vi "Select host address.vi"(0 "System number":i32=1 min=1 max=4 step=1, 1 "Port":i32=50000, 2 "Controller names":string[](array[string]), 3 "Mode":T1(ring), 4 "All?":bool, 5 "error in":errorcluster) -> (14 "Selected Host address/name":string="localhost", 15 "Port out":i32=50000, 19 "error out":errorcluster)   [LabVIEW 2026]
doc: "Performs an UDP broadcast, returns IP addresses and names of all controllers matching Controller name and lets the user select the appropriate controller from a ring control. VI will also stop if Cancel is TRUE.\n\nC-413: Controller names = C-413, Mode = Find XPort by UDP, Port = 30718\nC-413: Controller names = C-413, Mode = Find USR-K3 by UDP, Port = 1901\nC-702: Controller names = C-702, Mode = Find controller by UDP, Port = 50000 \nC-867: Controller names = C-867, Mode = Find controller by UDP, Port = 50000\nC-884: Controller names = C-884, Mode = Find controller by UDP, Port = 50000\nC-885: Controller names = C-885, Mode = Find controller by UDP, Port = 50000\nC-886: Controller names = C-886, Mode = Find controller by UDP, Port = 50000\nC-891: Controller names = C-891, Mode = Find XPort by UDP, Port = 30718\nE-135: Controller names = E-135, Mode = Find USR-K3 by UDP, Port = 1901\nE-517: Controller names = E-517, Mode = Find controller by UDP, Port = 50000\nE-518: Controller names = E-518, Mode = Find controller by UDP, Port = 50000\nE-712: Controller names = E-712, Mode = Find controller by UDP, Port = 50000\nE-725: Controller names = E-725, Mode = Find XPort by UDP, Port = 30718\nE-725: Controller names = E-725, Mode = Find controller by UDP, Port = 50000\nE-753: Controller names = E-753, Mode = Find controller by UDP, Port = 50000\nE-754: Controller names = E-754, Mode = Find controller by UDP, Port = 50000\nE-871: Controller names = E-871, Mode = Find XPort by UDP, Port = 30718\nE-872: Controller names = E-872, Mode = Find controller by UDP, Port = 50000\nE-873: Controller names = E-873, Mode = Find XPort by UDP, Port = 30718\nE-874: Controller names = E-874, Mode = Find USR-K3 by UDP, Port = 1901\nF-206: Controller names = F-206, F-HEX, Mode = Find XPort by UDP, Port = 30718\nC-887, M-8X0: Controller names = M-8X0, HEXAPOD, Mode = Find XPort by UDP, Port = 30718"
panel:
  in  "abort":bool
  in  "ok":bool
  in  "Please select controller":u16(ring) items=["(c)2013-2015 Physik Instrumente (PI) GmbH & Co. KG,C-413K006,0155500004,0.011 -- listening on port 2000 -- at address: 172.16.50.50"]
  out "Please wait":string="Broadcast is running, please wait..."
  # "Port to scan and controller name to search for:"
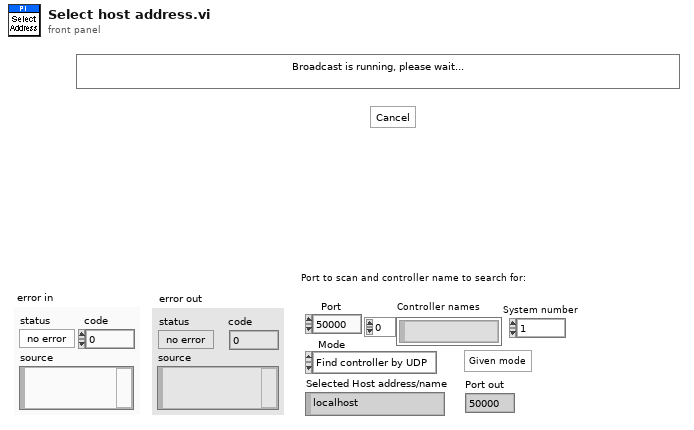
[diagram p1: front panel]
types:
  T1 = enum16{"Find controller by UDP", "Find XPort by UDP", "Find USR-K3 by UDP"}
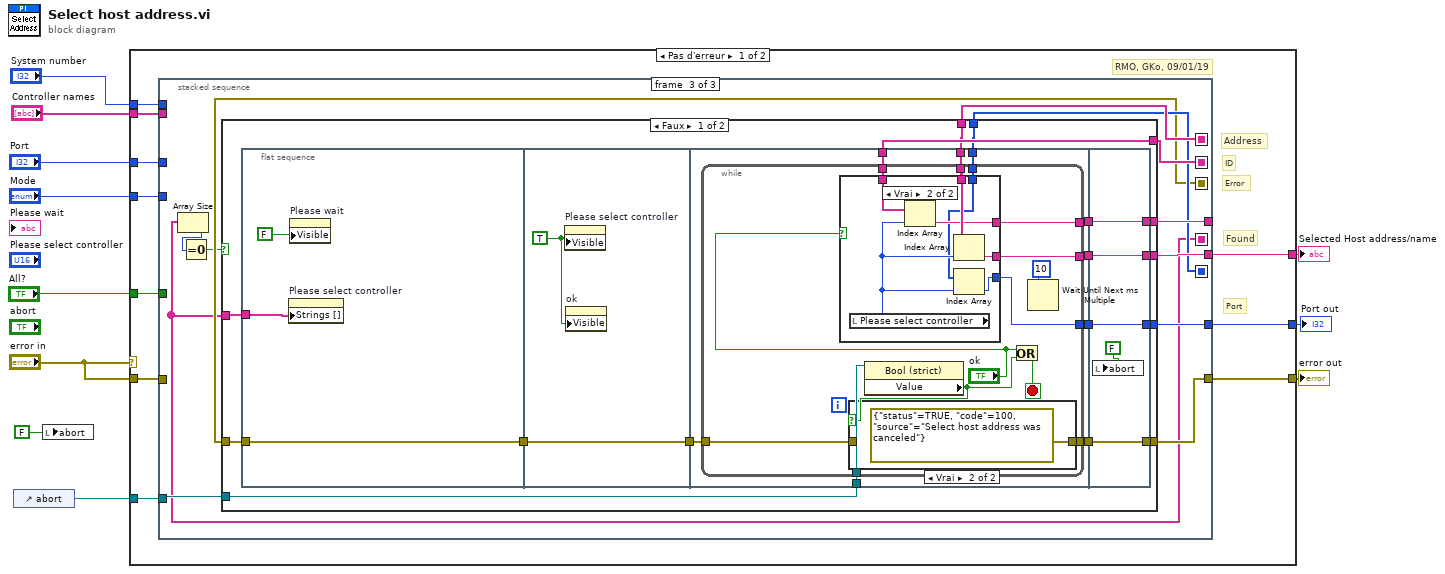
[diagram p0: block diagram]
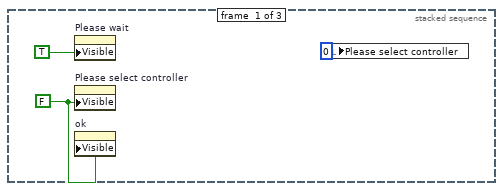
[diagram p2: hidden frame]
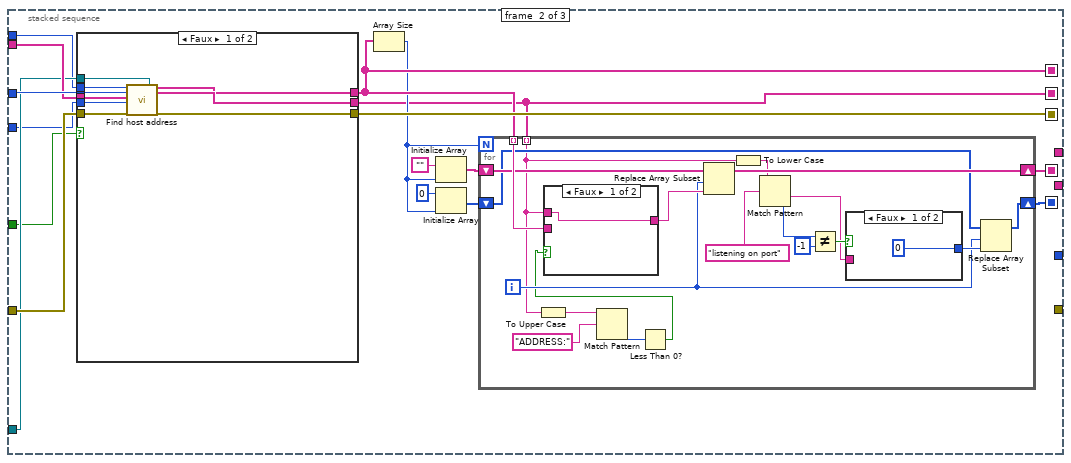
[diagram p3: hidden frame]
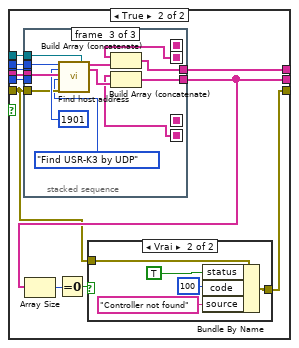
[diagram p4: hidden frame]
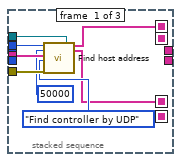
[diagram p6: hidden frame]
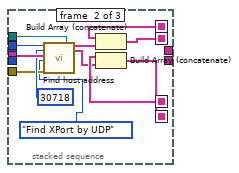
[diagram p7: hidden frame]
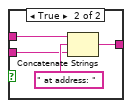
[diagram p8: hidden frame]
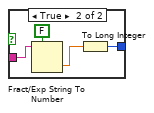
[diagram p9: hidden frame]
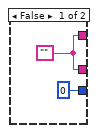
[diagram p11: hidden frame]
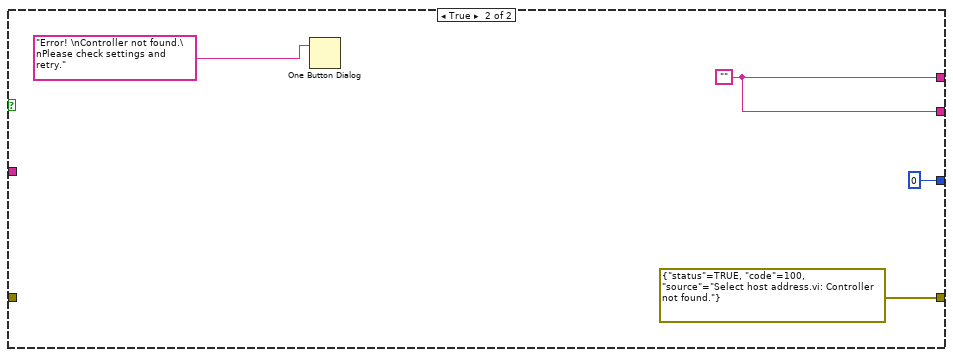
[diagram p12: hidden frame]
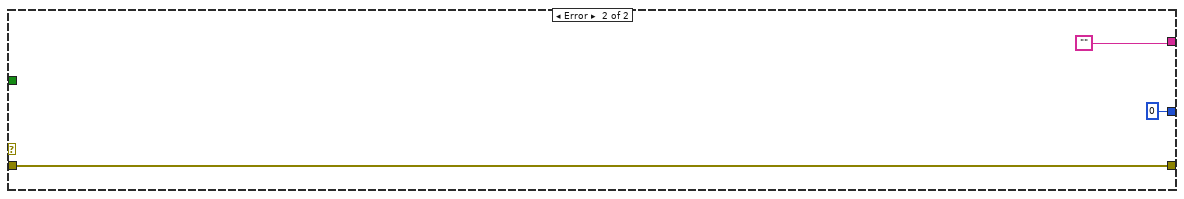
[diagram p13: hidden frame]
diagram:
  n1 = control-ref of="abort"() -> (w8:refnum<vi>)
  n2 = local write "abort"(FALSE ("abort")) -> ()
  n3 = case shown="Pas d'erreur" "error in" {
    tunnel: [w18 w206] -> w11
    tunnel: "error in" -> [w19 w206]
    tunnel: "Port" -> [w21 _]
    tunnel: "Controller names" -> [w20 _]
    tunnel: w8 -> [w17 _]
    tunnel: [w15 "" ("Host address/name")] -> w7
    tunnel: "Mode" -> [w16 _]
    tunnel: [w14 0] -> w5
    tunnel: "System number" -> [w13 _]
    tunnel: "All?" -> [w12 _]
    frame No Error {
      # "Port"
      # "Error"
      # "Found"
      # "Address"
      # "ID"
      # "RMO, GKo, 09/01/19"
      n4 = stacked-sequence {
        seq-local: [_ w36 _] -> [_ _ w133]
        seq-local: [_ w35 _] -> [_ _ w131]
        seq-local: [_ w34 _] -> [_ _ w139]
        seq-local: [_ w25 _] -> [_ _ w140]
        seq-local: [_ w28 _] -> [_ _ w135]
        tunnel: w21 -> [_ w41 _]
        tunnel: w20 -> [_ w40 _]
        tunnel: w19 -> [_ w39 _]
        tunnel: [_ _ w132] -> w18
        tunnel: [_ _ w138] -> _
        tunnel: [_ _ w137] -> w15
        tunnel: w17 -> [_ w33 w136]
        tunnel: w16 -> [_ w32 _]
        tunnel: [_ _ w134] -> w14
        tunnel: w13 -> [_ w27 _]
        tunnel: w12 -> [_ w26 _]
        frame #0 {
          w23 = FALSE ("Visible")
          n5 = property on="Please wait" class="Ch"("Visible"=TRUE) -> ()  [unwired: 2 in, 2 out]
          n6 = property on="Please select controller" class="MDér (strict)"("Visible"=w23) -> ()  [unwired: 2 in, 2 out]
          n7 = property on="ok" class="Bool"("Visible"=w23) -> ()  [unwired: 2 in, 2 out]
          n8 = local write "Please select controller"(0) -> ()
        }
        frame #1 {
          n9 = case shown="Faux" w26 {
            tunnel: w41 -> [w50 w61]
            tunnel: w40 -> [w49 w60]
            tunnel: w39 -> [w48 w51]
            tunnel: [w47 w53] -> w36
            tunnel: [w46 w52] -> w25
            tunnel: [w45 w59] -> w34
            tunnel: w33 -> [w44 w58]
            tunnel: w32 -> [w43 w57]
            tunnel: w27 -> [w42 w56]
            frame False {
              n10 = call "Find host address.vi"("System number"=w42, "Port"=w50, "Controller names"=w49, "Mode"=w43, "error in"=w48, "Stop refnum"=w44) -> ("Address"=w45:string[], "ID"=w46:string[], "error out"=w47:errorcluster)  [unwired: 11 out]
            }
            frame True {
              n11 = stacked-sequence {
                seq-local: [w69 _ _] -> [_ w83 _]
                seq-local: [w68 _ _] -> [_ w81 _]
                seq-local: [_ w79 _] -> [_ _ w92]
                seq-local: [_ w78 _] -> [_ _ w91]
                tunnel: w61 -> [_ _ _]
                tunnel: w60 -> [w75 w87 w99]
                tunnel: w51 -> [w74 w77 w89]
                tunnel: [_ _ w90] -> w52
                tunnel: [_ _ w94] -> w59
                tunnel: w58 -> [w73 w86 w98]
                tunnel: w57 -> [_ _ _]
                tunnel: w56 -> [w72 w85 w97]
                frame #0 {
                  n12 = call "Find host address.vi"("System number"=w72, "Port"=50000, "Controller names"=w75, "Mode"=T1."Find controller by UDP", "error in"=w74, "Stop refnum"=w73) -> ("Address"=w69:string[], "ID"=w68:string[])  [unwired: 12 out]
                }
                frame #1 {
                  n13 = call "Find host address.vi"("System number"=w85, "Port"=30718, "Controller names"=w87, "Mode"=T1."Find XPort by UDP", "error in"=w77, "Stop refnum"=w86) -> ("Address"=w82:string[], "ID"=w80:string[])  [unwired: 12 out]
                  n14 = Build Array (concatenate)(w83, w82) -> (w79:string[])
                  n15 = Build Array (concatenate)(w81, w80) -> (w78:string[])
                }
                frame #2 {
                  n16 = call "Find host address.vi"("System number"=w97, "Port"=1901, "Controller names"=w99, "Mode"=T1."Find USR-K3 by UDP", "error in"=w89, "Stop refnum"=w98) -> ("Address"=w95:string[], "ID"=w93:string[])  [unwired: 12 out]
                  n17 = Build Array (concatenate)(w92, w95) -> (w94:string[])
                  n18 = Build Array (concatenate)(w91, w93) -> (w90:string[])
                }
              }
              n19 = Array Size(array=w52) -> (size(s)=w54:i32)
              n20 = Equal To 0?(x=w54) -> (x = 0?=w55:bool)
              n21 = case shown="Vrai" w55 {
                tunnel: [w62 w64] -> w53
                tunnel: w51 -> [w62 w63]
                frame False {
                }
                frame True {
                  n22 = Bundle By Name(cluster=w63, "status"=TRUE, "code"=100 ("Bundle Element"), "source"="Controller not found" ("Bundle Element")) -> (w64:errorcluster)
                }
              }
            }
          }
          n23 = Array Size(array=w34) -> (size(s)=w30:i32)
          n24 = Initialize Array("", w30) -> (w38:string[])
          n25 = Initialize Array(0, w30) -> (w31:i32[])
          n26 = for {
            N: w30 -> [_]
            shift-right: [w115] -> w35
            shift-left: w38 -> [w117]
            tunnel: w25 -> [w104] mode=indexing
            tunnel: w34 -> [w118] mode=indexing
            shift-right: [w107] -> w28
            shift-left: w31 -> [w106]
            i -> [w108]
            n27 = To Upper Case(1:w104) -> (0:w103:string)
            n28 = Match Pattern(string=w103, regular expression="ADDRESS:") -> (offset past match=w101:i32)  [unwired: 4 out]
            n29 = Less Than 0?(x=w101) -> (x < 0?=w100:bool)
            n30 = case shown="Faux" w100 {
              tunnel: w118 -> [_ w122]
              tunnel: [w119 w121] -> w116
              tunnel: w104 -> [w119 w120]
              frame False {
              }
              frame True {
                n31 = Concatenate Strings(w120, " at address: ", w122) -> (w121:string)
              }
            }
            n32 = Replace Array Subset(array=w117, new element=w116, index=w108) -> (w115:string[])
            n33 = To Lower Case(string=w104) -> (all lower case string=w105:string)
            n34 = Match Pattern(string=w105, regular expression="listening on port") -> (after substring=w110:string, offset past match=w112:i32)  [unwired: 3 out]
            n35 = Not Equal?(x=w112, y=-1) -> (x != y?=w111:bool)
            n36 = case shown="Faux" w111 {
              tunnel: w110 -> [_ w127]
              tunnel: [0 w125] -> w109
              frame False {
              }
              frame True {
                n37 = Fract/Exp String To Number(use system decimal point (T)=FALSE, string=w127) -> (number=w126:dbl)  [unwired: 3 out]
                n38 = To Long Integer(number=w126) -> (32bit integer=w125:i32)
              }
            }
            n39 = Replace Array Subset(array=w106, new element=w109, index=w108) -> (w107:i32[])
          }
        }
        frame #2 {
          n40 = Array Size(array=w131) -> (size(s)=w130:i32)
          n41 = Equal To 0?(x=w130) -> (x = 0?=w129:bool)
          n42 = case shown="Faux" w129 {
            tunnel: w131 -> [w156 _]
            tunnel: w140 -> [w155 _]
            tunnel: w139 -> [w154 _]
            tunnel: [w153 w202] -> w138
            tunnel: [w152 w202] -> w137
            tunnel: w136 -> [w151 _]
            tunnel: w135 -> [w148 _]
            tunnel: [w147 0] -> w134
            tunnel: w133 -> [w145 _]
            tunnel: [w141 errorcluster {"status"=TRUE, "code"=100, "source"="Select host address.vi: Controller not found."} ("error out")] -> w132
            frame False {
              n43 = flat-sequence {
                tunnel: w156 -> [w158]
                tunnel: w145 -> [w157]
                tunnel: [w157] -> w144
                tunnel: w144 -> [w160]
                tunnel: [w160] -> w143
                tunnel: w155 -> [w170]
                tunnel: w154 -> [w169]
                tunnel: w151 -> [w166]
                tunnel: [w168] -> w150
                tunnel: [w167] -> w149
                tunnel: w148 -> [w165]
                tunnel: [w164] -> w146
                tunnel: w143 -> [w163]
                tunnel: [w162] -> w142
                tunnel: [w198] -> w152
                tunnel: [w199] -> w153
                tunnel: w150 -> [w199]
                tunnel: w149 -> [w198]
                tunnel: [w196] -> w147
                tunnel: w146 -> [w196]
                tunnel: [w195] -> w141
                tunnel: w142 -> [w195]
                frame #0 {
                  n44 = property on="Please select controller" class="MDér (strict)"("Strings []"=w158) -> ()  [unwired: 2 in, 2 out]
                  n45 = property on="Please wait" class="Ch"("Visible"=FALSE) -> ()  [unwired: 2 in, 2 out]
                }
                frame #1 {
                  w161 = TRUE ("Visible")
                  n46 = property on="Please select controller" class="MDér (strict)"("Visible"=w161) -> ()  [unwired: 2 in, 2 out]
                  n47 = property on="ok" class="Bool"("Visible"=w161) -> ()  [unwired: 2 in, 2 out]
                }
                frame #2 {
                  n48 = while {
                    tunnel: w170 -> [w181]
                    tunnel: w169 -> [w180]
                    tunnel: [w179] -> w168
                    tunnel: [w178] -> w167
                    tunnel: w166 -> [w177]
                    tunnel: w165 -> [w176]
                    tunnel: [w175] -> w164
                    tunnel: w163 -> [w174]
                    tunnel: [w173] -> w162
                    stop <- w183 stop-if-true
                    n49 = case shown="Vrai" "ok" {
                      tunnel: w181 -> [_ w194]
                      tunnel: w180 -> [_ w193]
                      tunnel: [w187 w192] -> w179
                      tunnel: [w187 w191] -> w178
                      tunnel: w176 -> [_ w189]
                      tunnel: [0 w188] -> w175
                      frame False {
                        w187 = "" ("Host address/name")
                      }
                      frame True {
                        n50 = local read "Please select controller"() -> (w190:u16)
                        n51 = Index Array(array=w194, index=w190) -> (element=w192:string)
                        n52 = Index Array(array=w193, index=w190) -> (element=w191:string)
                        n53 = Index Array(array=w189, index=w190) -> (element=w188:i32)
                      }
                    }
                    n54 = property class="Bool (strict)"(reference=w177) -> ("Value"=w172:bool)  [unwired: 1 in, 2 out]
                    n55 = case shown="Vrai" w172 {
                      tunnel: w174 -> [w184 _]
                      tunnel: [w184 errorcluster {"status"=TRUE, "code"=100, "source"="Select host address was canceled"} ("error out")] -> w173
                      frame False {
                      }
                      frame True {
                      }
                    }
                    n56 = Or(x="ok", y=w172) -> (x .or. y?=w183:bool)
                    n57 = Wait Until Next ms Multiple(millisecond multiple=u32 10) -> ()  [unwired: 1 out]
                  }
                }
                frame #3 {
                  n58 = local write "abort"(FALSE ("abort")) -> ()
                }
              }
            }
            frame True {
              w202 = "" ("Host address/name")
              n59 = One Button Dialog(message="Error! \nController not found.\nPlease check settings and retry.") -> ()  [unwired: 2 out]
            }
          }
        }
      }
    }
    frame Error {
    }
  }
  "error out" <- w11
  "Selected Host address/name" <- w7
  "Port out" <- w5
